vi "Data To SingleElementsArray.vi"(8 "error in (no error)":errorcluster, 10 "parentUrl":string, 11 "Cluster":variant) -> (0 "error out":errorcluster, 1 "Tree Discription":string[][](array[string]), 2 "Full NameList":string[](array[string]), 3 "DataElementArray":variant[](array[variant]))   [LabVIEW 2017]
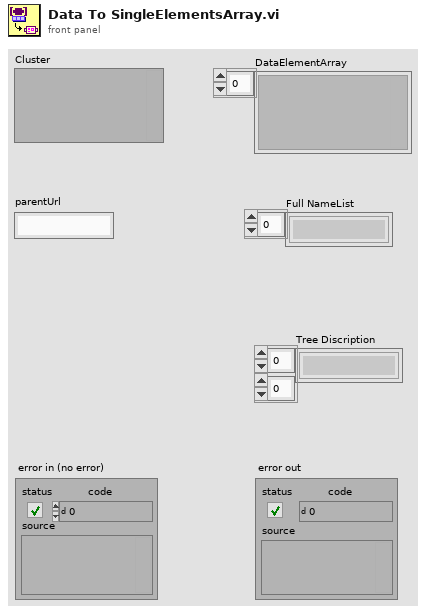
[diagram p1: front panel]
types:
  T1 = typedef "Type Descriptor Enumeration__ogtk.ctl" = enum8{"<Null>", "I8", "I16", "I32", "I64", "U8", "U16", "U32", "U64", "SGL", "DBL", "EXT", "CSG", "CDB", "CXT", "0x0F", "0x10", "0x11", "0x12", "0x13", "0x14", "Enum U8", "Enum U16", "Enum U32", "Enum U64", "SGL PQ", "DBL PQ", "EXT PQ", "CSG PQ", "CDB PQ", "CXT PQ", "0x1F", "0x20", "Boolean", "0x22", "0x23", "0x24", "0x25", "0x26", "0x27", "0x28", "0x29", "0x2A", "0x2B", "0x2C", "0x2D", "0x2E", "0x2F", "String", "0x31", "Path", "Pict", "0x34", "0x35", "0x36", "DAQ", "0x38", "0x39", "0x3A", "0x3B", "0x3C", "0x3D", "0x3E", "0x3F", "Array", "0x41", "0x42", "0x43", "0x44", "0x45", "0x46", "0x47", "0x48", "0x49", "0x4A", "0x4B", "0x4C", "0x4D", "0x4E", "0x4F", "Cluster", "0x51", "0x52", "Variant", "Waveform", "0x55", "0x56", "0x57", "0x58", "0x59", "0x5A", "0x5B", "0x5C", "0x5D", "0x5E", "0x5F", "0x60", "0x61", "0x62", "0x63", "0x64", "0x65", "0x66", "0x67", "0x68", "0x69", "0x6A", "0x6B", "0x6C", "0x6D", "0x6E", "0x6F", "Refnum"}
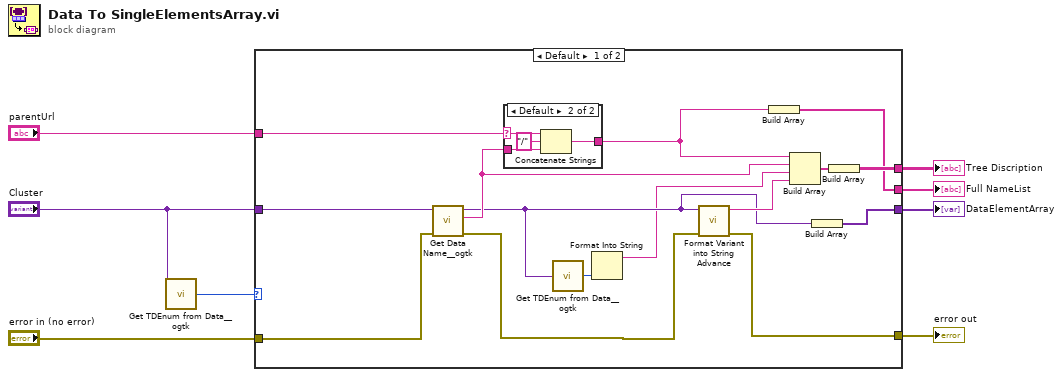
[diagram p0: block diagram]
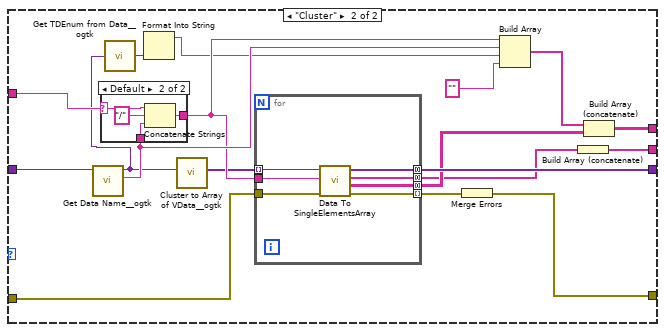
[diagram p3: hidden frame]
diagram:
  n1 = call <userlib>:"Get TDEnum from Data__ogtk.vi"("Data"="Cluster") -> ("Type Descriptor Enumeration"=w8:T1)  [unwired: 4 in]
  n2 = case shown="Default" w8 {
    tunnel: "Cluster" -> [w23 w46]
    tunnel: "parentUrl" -> [w22 w42]
    tunnel: [w15 w39] -> w2
    tunnel: "error in (no error)" -> [w18 w45]
    tunnel: [w17 w43] -> w4
    tunnel: [w16 w35] -> w3
    tunnel: [w13 w32] -> w1
    frame Default {
      n3 = call <userlib>:"Get Data Name__ogtk.vi"("error in (no error)"=w18, "Data"=w23) -> ("error out"=w12:errorcluster, "Data Name"=w21:string, "Data dup"=w10:variant)  [unwired: 7 in]
      n4 = case shown="Default" w22 {
        selector: w22 -> [_ w28]
        tunnel: [w24 w26] -> w14
        tunnel: w21 -> [w24 w25]
        frame "" {
        }
        frame Default {
          n5 = Concatenate Strings(w28, "/" ("element"), w25) -> (w26:string)
        }
      }
      n6 = call <userlib>:"Get TDEnum from Data__ogtk.vi"("Data"=w10) -> ("Type Descriptor Enumeration"=w11:T1)  [unwired: 4 in]
      n7 = Format Into String(w11) -> (resulting string=w9:string)  [unwired: 3 in, 1 out]
      n8 = call "Format Variant into String Advance.vi"("error in (no error)"=w12, "Variant"=w10) -> ("error out"=w17:errorcluster, "Data"=w20:string)  [unwired: 7 in, 1 out]
      n9 = Build Array(w14) -> (w13:string[])
      n10 = Build Array(w14, w21, w9, w20) -> (w19:string[])
      n11 = Build Array(w10) -> (w16:variant[])
      n12 = Build Array(w19) -> (w15:string[][])
    }
    frame "Cluster" {
      n13 = call <userlib>:"Get Data Name__ogtk.vi"("Data"=w46) -> ("Data Name"=w41:string, "Data dup"=w31:variant)  [unwired: 8 in, 1 out]
      n14 = case shown="Default" w42 {
        selector: w42 -> [_ w49]
        tunnel: w41 -> [w47 w50]
        tunnel: [w47 w48] -> w37
        frame "" {
        }
        frame Default {
          n15 = Concatenate Strings(w49, "/" ("element"), w50) -> (w48:string)
        }
      }
      n16 = call <userlib>:"Get TDEnum from Data__ogtk.vi"("Data"=w31) -> ("Type Descriptor Enumeration"=w30:T1)  [unwired: 4 in]
      n17 = Format Into String(w30) -> (resulting string=w29:string)  [unwired: 3 in, 1 out]
      n18 = call <userlib>:"Cluster to Array of VData__ogtk.vi"("Cluster"=w31) -> ("Array of VData"=w36:variant[])  [unwired: 9 in, 1 out]
      n19 = for {
        tunnel: w36 -> [w58] mode=indexing
        tunnel: w37 -> [w57]
        tunnel: [w56] -> w35 mode=concatenating
        tunnel: w45 -> [w55]
        tunnel: [w54] -> w44 mode=indexing
        tunnel: [w53] -> w34 mode=concatenating
        tunnel: [w52] -> w33 mode=concatenating
        n20 = call "Data To SingleElementsArray.vi"("error in (no error)"=w55, "parentUrl"=w57, "Cluster"=w58) -> ("error out"=w54:errorcluster, "Tree Discription"=w53:string[][], "Full NameList"=w52:string[], "DataElementArray"=w56:variant[])  [unwired: 5 in]
      }
      n21 = Merge Errors(w44) -> (w43:errorcluster)
      n22 = Build Array(w37, w41, w29, "" ("element")) -> (w38:string[])
      n23 = Build Array (concatenate)(w33) -> (w32:string[])
      n24 = Build Array (concatenate)(w38, w34) -> (w39:string[][])
    }
  }
  "Full NameList" <- w1
  "error out" <- w4
  "DataElementArray" <- w3
  "Tree Discription" <- w2
